vi "题目六.vi"   [LabVIEW 2017]
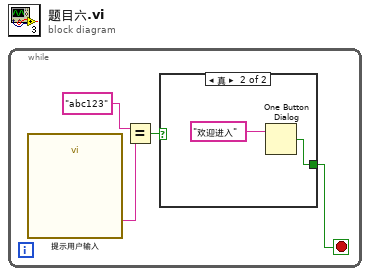
[diagram p0: block diagram]
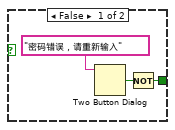
[diagram p2: hidden frame]
diagram:
  n1 = while {
    stop <- w1 stop-if-true
    n2 = call "提示用户输入"() -> ("输入密码"=w4:string)  [unwired: 17 in, 2 out]
    n3 = Equal?(x="abc123", y=w4) -> (x = y?=w2:bool)
    n4 = case shown="真" w2 {
      tunnel: [w5 w8] -> w1
      frame False {
        n5 = Two Button Dialog(message="密码错误，请重新输入") -> (T button?=w6:bool)  [unwired: 2 in]
        n6 = Not(x=w6) -> (.not. x?=w5:bool)
      }
      frame True {
        n7 = One Button Dialog(message="欢迎进入") -> (true=w8:bool)  [unwired: 1 in]
      }
    }
  }
